vi "Read List of Measurements.vi"(8 "error in (no error)":errorcluster, 11 "List of Measurements Message in":refnum<class "List of Measurements Message.lvclass">) -> (0 "error out":errorcluster, 2 "List of Measurements":string[](array[string]), 3 "List of Measurements Message out":refnum<class "List of Measurements Message.lvclass">)   [LabVIEW 2016, in "Controller UI.lvlib" / "List of Measurements Message.lvclass"]
uses:
  <userlib>/Common Components/Controller UI/Messages/List of Measurements Message/List of Measurements Message.lvclass
  <userlib>/Common Components/Controller UI/Messages/List of Measurements Message/List of Measurements Message.lvclass/List of Measurements Message.ctl
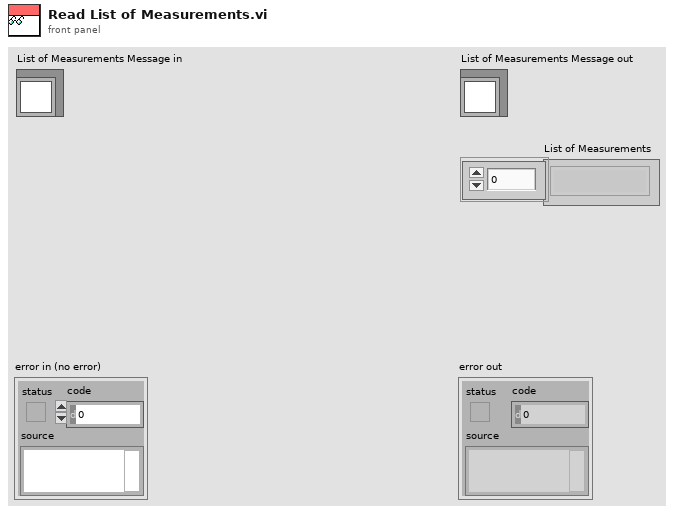
[diagram p1: front panel]
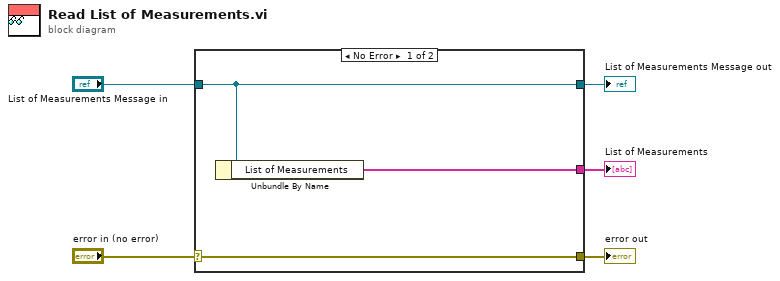
[diagram p0: block diagram]
diagram:
  n1 = case shown="No Error" "error in (no error)" {
    selector: "error in (no error)" -> [w8 w9]
    tunnel: [w8 w9] -> w4
    tunnel: [w7 w10] -> w2
    tunnel: "List of Measurements Message in" -> [w7 w10]
    tunnel: [w6 _] -> w1
    frame No Error {
      n2 = Unbundle By Name(w7) -> ("List of Measurements"=w6:string[])
    }
    frame Error {
    }
  }
  "error out" <- w4
  "List of Measurements Message out" <- w2
  "List of Measurements" <- w1
